vi "Sort Cluster.vi"(8 "error in (no error)":errorcluster, 11 "Array in":T1[](array[typedef])) -> (0 "error out":errorcluster, 3 "Array out":T1[](array[typedef]))   [LabVIEW 2025, in "Project.lvclass"]
doc: "Sort signals under a given FPGA target and under a given module by IO Resource"
uses:
  Project.lvclass
  FPGA Settings.ctl
  Module/Module/Module Settings.ctl
  Signal/Signal/Signal Settings.ctl
  Project.lvclass/Project.ctl
  Signal/Signal/Signal.lvclass
  Module/Module/Module.lvclass
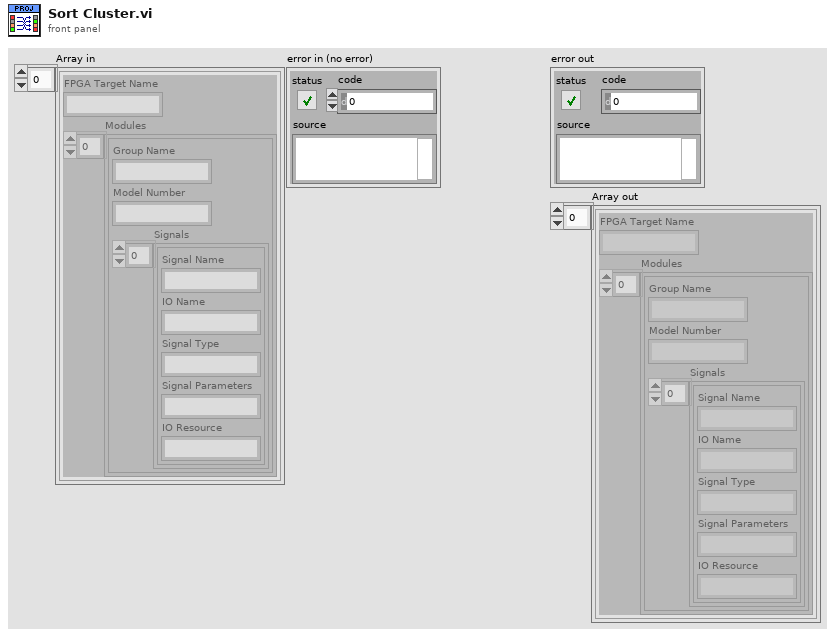
[diagram p1: front panel]
types:
  T1 = typedef "Project.lvclass/FPGA Settings.ctl" = cluster{"FPGA Target Name":string, "Modules":T2[]}
  T2 = typedef "Module.lvclass/Module Settings.ctl" = cluster{"Group Name":string, "Model Number":string, "Signals":T3[]}
  T3 = typedef "Signal.lvclass/Signal Settings.ctl" = cluster{"Signal Name":string, "IO Name":string, "Signal Type":string, "Signal Parameters":string, "IO Resource":string}
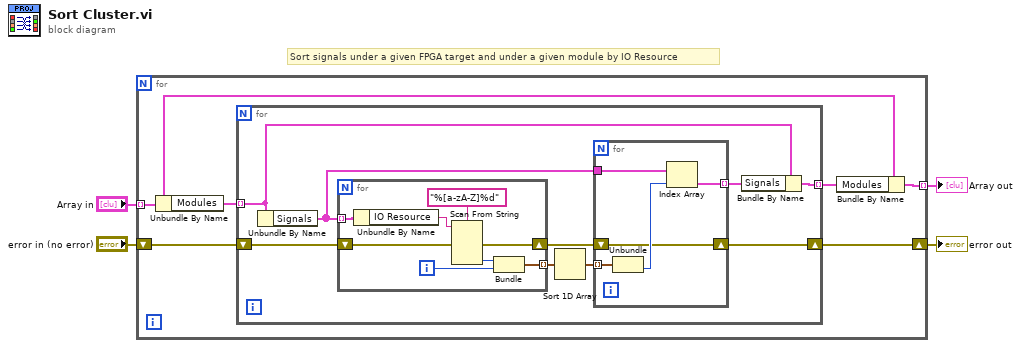
[diagram p0: block diagram]
diagram:
  # "Sort signals under a given FPGA target and under a given module by IO Resource"
  n1 = for {
    tunnel: "Array in" -> [w7] mode=indexing
    shift-right: [w8] -> w2
    shift-left: "error in (no error)" -> [w9]
    tunnel: [w5] -> w1 mode=indexing
    n2 = Unbundle By Name(w7) -> ("Modules"=w10:T2[])
    n3 = for {
      tunnel: w10 -> [w13] mode=indexing
      shift-right: [w14] -> w8
      shift-left: w9 -> [w16]
      tunnel: [w11] -> w6 mode=indexing
      n4 = Unbundle By Name(w13) -> ("Signals"=w17:T3[])
      n5 = for {
        tunnel: w17 -> [w32] mode=indexing
        tunnel: [w27] -> w19 mode=indexing
        shift-right: [w25] -> w15
        shift-left: w16 -> [w26]
        i -> [w28]
        n6 = Unbundle By Name(w32) -> ("IO Resource"=w30:string)
        n7 = Scan From String(format string="%[a-zA-Z]%d", input string=w30, error in=w26) -> (error out=w25:errorcluster, output 2=w29:i32)  [unwired: 4 in, 2 out]
        n8 = Bundle(w29, w28) -> (w27:cluster{i32, i32})  [unwired: 1 in]
      }
      n9 = Sort 1D Array(array=w19) -> (sorted array=w18:cluster{i32, i32}[])
      n10 = for {
        tunnel: w18 -> [w24] mode=indexing
        tunnel: w17 -> [w22]
        shift-right: [w21] -> w14
        shift-left: w15 -> [w21]
        tunnel: [w20] -> w12 mode=indexing
        n11 = Unbundle(w24) -> (w23:i32)  [unwired: 1 out]
        n12 = Index Array(array=w22, index=w23) -> (element=w20:T3)
      }
      n13 = Bundle By Name(cluster=w13, "Signals"=w12) -> (w11:T2)
    }
    n14 = Bundle By Name(cluster=w7, "Modules"=w6) -> (w5:T1)
  }
  "error out" <- w2
  "Array out" <- w1
